vi "Delete Int8Array DVR.vi"(8 "error in (no error)":errorcluster, 11 "Int8Array DVR in":refnum<data-value>) -> (0 "error out":errorcluster, 3 "Int8Array out":refnum<class "Int8Array.lvclass">)   [LabVIEW 2012, in "MDSplus.lvlib" / "Int8Array.lvclass"]
uses:
  <vilib>/MDSplus/Classes/Data_Class/Array_Class/Int8Array_Class/Int8Array.lvclass
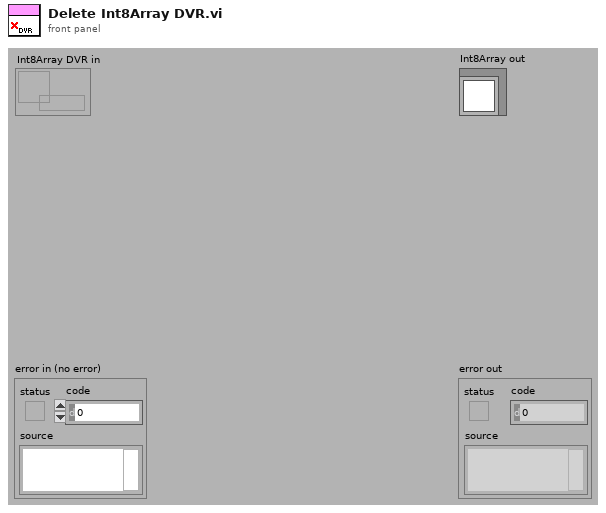
[diagram p1: front panel]
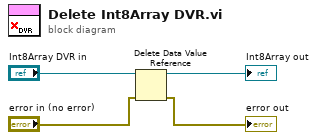
[diagram p0: block diagram]
diagram:
  n1 = Delete Data Value Reference(data value reference="Int8Array DVR in", error in="error in (no error)") -> (data value=→"Int8Array out":refnum<class "Int8Array.lvclass">, error out=→"error out":errorcluster)
